vi "MCP2221_GetGpioValues.vi"(8 "error in":errorcluster, 9 "handle in":i32) -> (0 "error out":errorcluster, 1 "handle out":i32, 2 "gpio":bool[](array[boolean]), 3 "return type":i32)   [LabVIEW 2025]
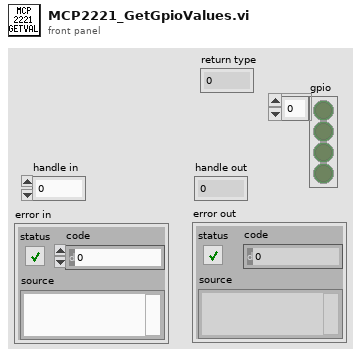
[diagram p1: front panel]
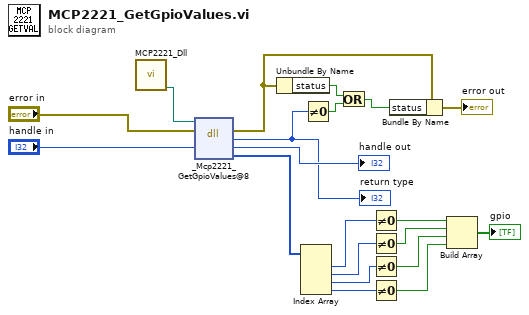
[diagram p0: block diagram]
diagram:
  n1 = call "MCP2221_Dll.vi"() -> ("dll path"=w17:path)  [unwired: 11 in]
  n2 = dll-call lib="?" fn="_Mcp2221_GetGpioValues@8"(path in=w17, error in="error in", "handle"="handle in") -> (error out=w13:errorcluster, "return type"=w12:i32, "handle"=→"handle out":i32, "gpio"=w6:u8[])  [unwired: 2 in, 1 out]
  "return type" <- w12
  n3 = Unbundle By Name(w13) -> ("status"=w16:bool)
  n4 = Index Array(array=w6) -> (element #1=w10:u8, element #2=w9:u8, element #3=w8:u8, element #4=w7:u8)  [unwired: 4 in]
  n5 = Not Equal To 0?(x=w12) -> (x != 0?=w14:bool)
  n6 = Or(x=w16, y=w14) -> (x .or. y?=w15:bool)
  n7 = Not Equal To 0?(x=w10) -> (x != 0?=w5:bool)
  n8 = Not Equal To 0?(x=w9) -> (x != 0?=w4:bool)
  n9 = Not Equal To 0?(x=w8) -> (x != 0?=w3:bool)
  n10 = Not Equal To 0?(x=w7) -> (x != 0?=w2:bool)
  n11 = Bundle By Name(cluster=w13, "status"=w15) -> (→"error out":errorcluster)
  n12 = Build Array(w5, w4, w3, w2) -> (→"gpio":bool[])
